vi "Read Type.vi"(8 "error in (no error)":errorcluster, 11 "PLC_Module in":refnum<class "PLC_Module.lvclass">) -> (0 "error out":errorcluster, 2 "Type":T1, 3 "PLC_Module out":refnum<class "PLC_Module.lvclass">)   [LabVIEW 2025, in "PLC_Module.lvlib" / "PLC_Module.lvclass"]
uses:
  PLC_Module.lvclass
  PLC_Module.lvclass/PLC_Module.ctl
  PLC_Type.ctl
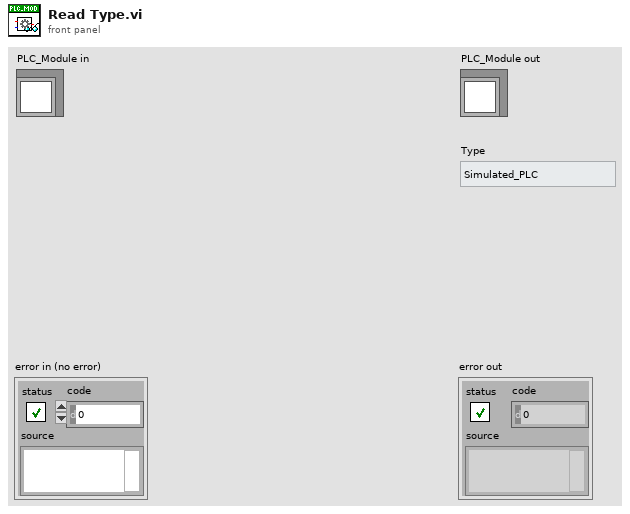
[diagram p1: front panel]
types:
  T1 = typedef "PLC_Module.lvlib/PLC_Module.lvclass/PLC_Type.ctl" = enum16{"Simulated_PLC", "SIMATIC_S7"}
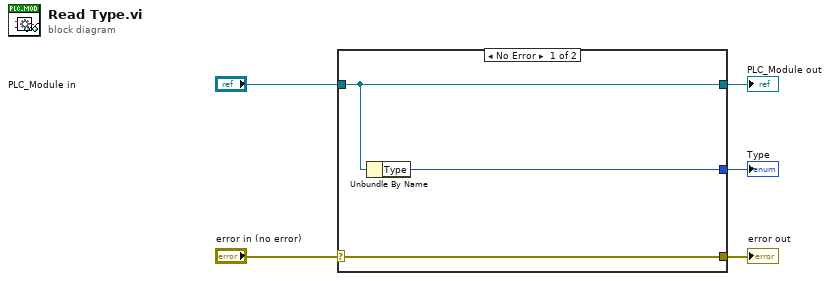
[diagram p0: block diagram]
diagram:
  n1 = case shown="No Error" "error in (no error)" {
    selector: "error in (no error)" -> [w8 w9]
    tunnel: [w8 w9] -> w4
    tunnel: [w7 w10] -> w2
    tunnel: "PLC_Module in" -> [w7 w10]
    tunnel: [w6 _] -> w1
    frame No Error {
      n2 = Unbundle By Name(w7) -> ("Type"=w6:T1)
    }
    frame Error {
    }
  }
  "error out" <- w4
  "PLC_Module out" <- w2
  "Type" <- w1
